vi "Set All Attributes.vi"(8 "error in":errorcluster, 10 "Channel Node":refnum<k20>, 11 "Channel Ref in":refnum<data-value>) -> (0 "error out":errorcluster, 3 "Channel Ref out":refnum<data-value>)   [LabVIEW 2024, in "Config File Parser.lvlib" / "Channel.lvclass"]
uses:
  Channel.lvclass
  Channel.lvclass/Channel.ctl
  <vilib>/xml/Close Reference(Node).vi
  <resource>/objmgr/DOMUserDefRef.rc
  <vilib>/xml/NI_XML.lvlib
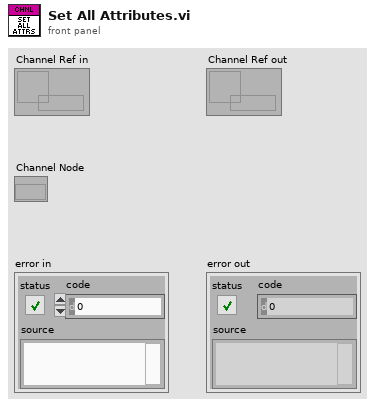
[diagram p1: front panel]
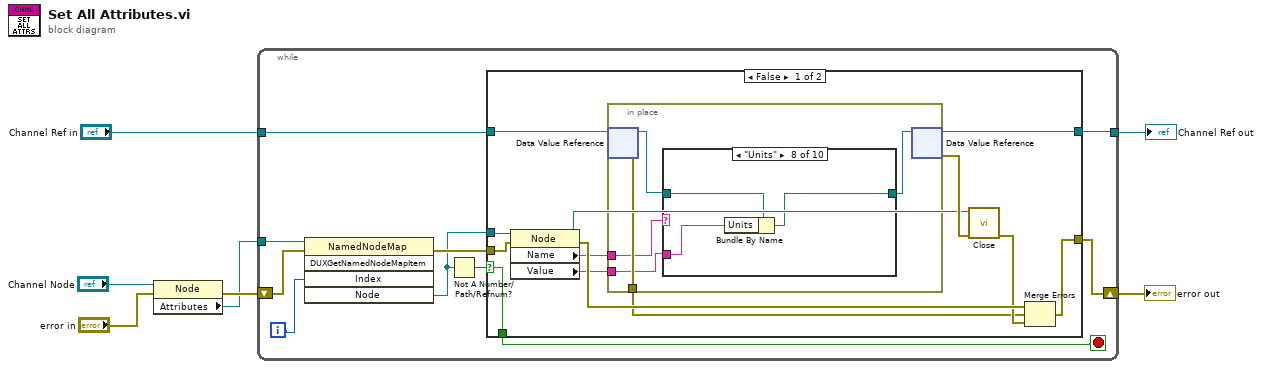
[diagram p0: block diagram]
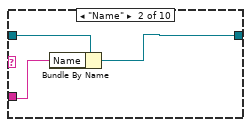
[diagram p3: hidden frame]
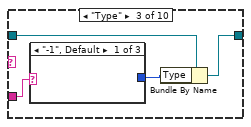
[diagram p4: hidden frame]
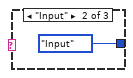
[diagram p5: hidden frame]
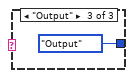
[diagram p6: hidden frame]
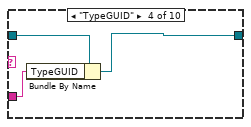
[diagram p7: hidden frame]
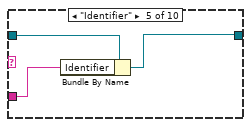
[diagram p8: hidden frame]
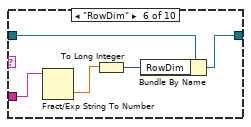
[diagram p9: hidden frame]
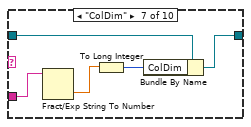
[diagram p10: hidden frame]
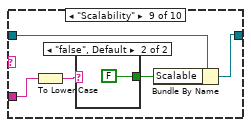
[diagram p11: hidden frame]
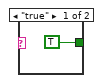
[diagram p12: hidden frame]
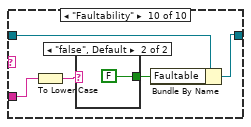
[diagram p13: hidden frame]
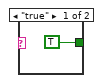
[diagram p14: hidden frame]
diagram:
  n1 = property on="Property Node" class="Node"(reference="Channel Node", error in="error in") -> (error out=w6:errorcluster, "Attributes"=w3:refnum<k20>)  [unwired: 1 out]
  n2 = while {
    tunnel: w3 -> [w14]
    shift-right: [w15] -> w5
    shift-left: w6 -> [w17]
    tunnel: "Channel Ref in" -> [w12]
    tunnel: [w10] -> w1
    i -> [w9]
    stop <- w8 stop-if-true
    n3 = invoke on="Invoke Node" class="NamedNodeMap" method="DUXGetNamedNodeMapItem"(reference=w14, error in=w17, "Index"=w9) -> (error out=w16:errorcluster, "Node"=w11:refnum<k20>)  [unwired: 2 in, 3 out]
    n4 = Not A Number/Path/Refnum?(number/path/refnum=w11) -> (NaN/Path/Refnum?=w13:bool)
    n5 = case shown="False" w13 {
      selector: w13 -> [w19 w79]
      tunnel: w12 -> [w21 w80]
      tunnel: w11 -> [w24 _]
      tunnel: w16 -> [w30 w81]
      tunnel: [w29 w81] -> w15
      tunnel: [w20 w80] -> w10
      tunnel: [w19 w79] -> w8
      frame False {
        n6 = property on="Property Node" class="Node"(reference=w24, error in=w30) -> (reference out=w22:refnum<k20>, error out=w28:errorcluster, "Name"=w23:string, "Value"=w18:string)
        n7 = in-place "In Place Element Structure" {
          in-place-border: w23 -> [w32]
          in-place-border: w18 -> [w31]
          in-place-border: [w35] -> w25
          n8 = in-place-dvr #1(w21) -> (w34:refnum<class "Channel.lvclass">, w35:errorcluster)
          n9 = case shown="\"Units\"" w32 {
            tunnel: w34 -> [w36 w38 w43 w47 w50 w56 w61 w63 w69 w76]
            tunnel: [w36 w37 w42 w46 w49 w55 w60 w62 w68 w75] -> w33
            tunnel: w31 -> [_ w39 w41 w48 w51 w54 w59 w64 w67 w74]
            frame "-1", Default {
            }
            frame "Name" {
              n10 = Bundle By Name(cluster=w38, "Name"=w39) -> (w37:refnum<class "Channel.lvclass">)
            }
            frame "Type" {
              n11 = case shown="\"-1\", Default" w41 {
                tunnel: [_ enum16{"Input", "Output"}."Input" enum16{"Input", "Output"}."Output"] -> w40
                frame "-1", Default {
                }
                frame "Input" {
                }
                frame "Output" {
                }
              }
              n12 = Bundle By Name(cluster=w43, "Type"=w40) -> (w42:refnum<class "Channel.lvclass">)
            }
            frame "TypeGUID" {
              n13 = Bundle By Name(cluster=w47, "TypeGUID"=w48) -> (w46:refnum<class "Channel.lvclass">)
            }
            frame "Identifier" {
              n14 = Bundle By Name(cluster=w50, "Identifier"=w51) -> (w49:refnum<class "Channel.lvclass">)
            }
            frame "RowDim" {
              n15 = Fract/Exp String To Number(string=w54) -> (number=w52:dbl)  [unwired: 3 in, 1 out]
              n16 = To Long Integer(number=w52) -> (32bit integer=w53:i32)
              n17 = Bundle By Name(cluster=w56, "RowDim"=w53) -> (w55:refnum<class "Channel.lvclass">)
            }
            frame "ColDim" {
              n18 = Fract/Exp String To Number(string=w59) -> (number=w57:dbl)  [unwired: 3 in, 1 out]
              n19 = To Long Integer(number=w57) -> (32bit integer=w58:i32)
              n20 = Bundle By Name(cluster=w61, "ColDim"=w58) -> (w60:refnum<class "Channel.lvclass">)
            }
            frame "Units" {
              n21 = Bundle By Name(cluster=w63, "Units"=w64) -> (w62:refnum<class "Channel.lvclass">)
            }
            frame "Scalability" {
              n22 = To Lower Case(string=w67) -> (all lower case string=w66:string)
              n23 = case shown="\"false\", Default" w66 {
                tunnel: [TRUE ("Scalability") FALSE ("Scalability")] -> w65
                frame "true" {
                }
                frame "false", Default {
                }
              }
              n24 = Bundle By Name(cluster=w69, "Scalable"=w65) -> (w68:refnum<class "Channel.lvclass">)
            }
            frame "Faultability" {
              n25 = To Lower Case(string=w74) -> (all lower case string=w73:string)
              n26 = case shown="\"false\", Default" w73 {
                tunnel: [TRUE ("Scalability") FALSE ("Scalability")] -> w72
                frame "true" {
                }
                frame "false", Default {
                }
              }
              n27 = Bundle By Name(cluster=w76, "Faultable"=w72) -> (w75:refnum<class "Channel.lvclass">)
            }
          }
          n28 = in-place-dvr #1(w33) -> (w20:refnum<data-value>, w27:errorcluster)
        }
        n29 = call-poly <vilib>:"Close.vi"("error in (no error)"=w27, "node"=w22) -> ("error out"=w26:errorcluster)  [unwired: 7 in]
        n30 = Merge Errors(w28, w25, w26) -> (w29:errorcluster)
      }
      frame True {
      }
    }
  }
  "error out" <- w5
  "Channel Ref out" <- w1
